vi "Destroy.vi"(0 "reference in":refnum<class "G#BaseClass2_IG#BaseInterface.lvclass">, 5 "error in (no error)":errorcluster) -> (14 "reference out":refnum<class "G#BaseClass2_IG#BaseInterface.lvclass">, 19 "error out":errorcluster)   [LabVIEW 2017, in "G#BaseClass2_IG#BaseInterface.lvclass"]
doc: "Destructor."
uses:
  G#BaseClass2_IG#BaseInterface.lvclass
  IG#BaseInterface_interface/IG#BaseInterface.lvclass
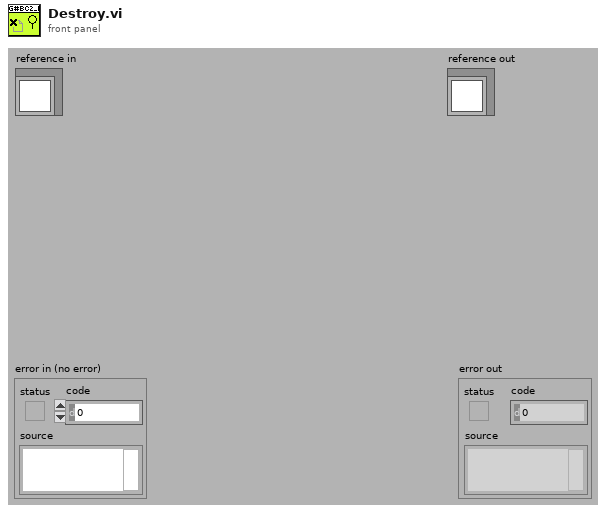
[diagram p1: front panel]
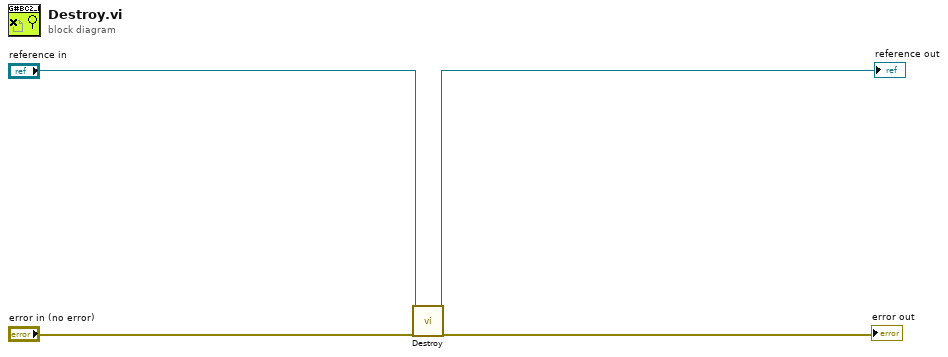
[diagram p0: block diagram]
diagram:
  n1 = call-parent "Destroy.vi"("reference in"="reference in", "error in (no error)"="error in (no error)") -> ("reference out"=→"reference out":refnum<class "G#BaseClass2_IG#BaseInterface.lvclass">, "error out"=→"error out":errorcluster)  [unwired: 16 in]
